vi "File Read Matrix.vi"(0 "file path (dialog if empty)":path, 11 "error in (no error)":errorcluster) -> (4 "Matrix":dbl[][](array[numeric]), 6 "Row Names":string[](array[string])=["AMP01BH", "AMP02AH", "AMP02BH", "AMP03AH", "AMP03BH", "AMP03CH", "AMP04AH", "AMP04BH", "AMP05AH", "AMP05BH", "AMP06AH", "AMP06BH", "AMP07AH", "AMP07BH", "AMP08AH", "AMP08BH", "AMP09AH", "AMP09BH", "AMP10AH", "AMP10BH", "AMU11AH", "AMU11BH", "AMP12AH", "AMP12BH", "AMP01AH", "AMP01BV", "AMP02AV", "AMP02BV", "AMP03AV", "AMP03BV", "AMP03CV", "AMP04AV", "AMP04BV", "AMP05AV", "AMP05BV", "AMP06AV", "AMP06BV", "AMP07AV", "AMP07BV", "AMP08AV", "AMP08BV", "AMP09AV", "AMP09BV", "AMP10AV", "AMP10BV", "AMU11AV", "AMU11BV", "AMP12AV", "AMP12BV", "AMP01AV"], 8 "Column Names":string[](array[string])=["ACH01B", "ACH02", "ACH03A", "ACH03B", "ACH04", "ACH05A", "ACH05B", "ACH06", "ACH07A", "ACH07B", "ACH08", "ACH09A", "ACH09B", "ACH10", "ACH11A", "ACH11B", "ACH12", "ACH01A", "ACV01B", "ALV02A", "ALV02B", "ACV03A", "ACV03B", "ALV04A", "ALV04B", "ACV05A", "ACV05B", "ALV06A", "ALV06B", "ACV07A", "ACV07B", "ALV08A", "ALV08B", "ACV09A", "ACV09B", "ALV10A", "ALV10B", "ACV11A", "ACV11B", "ALV12A", "ALV12B", "ACV01A"], 14 "Beam Energy (MeV)":dbl, 15 "error out":errorcluster)   [LabVIEW 2011, in "File VIs.lvlib"]
doc: "Reads a \"Response Matrix\" or \"Correction Matrix\" text file and converts the data to a 2D, double-precision array of numbers.\n\nFile format:\nFirst row: Beam Energy (MeV):<TAB>[Beam Energy Value for which the matrix was measured/calculated]\nSecond row*: Column names (Corrector names, for Response Matrix; BPM names, for Correction Matrix)\nAll other rows:\n Column 1: BPM names\n All other columns: Matrix value (mm/A, for Response Matrix; A/mm, for Correction Matrix)\nColumn separator: <TAB> character\n\n* The second row must begin with a <TAB> character\n\nEx.:\nBeam Energy (MeV):<TAB>1370\n<TAB>ACH01B<TAB>ACH02\nAMP01BH<TAB>5.10765701<TAB>-1.50432895\nAMP02AH<TAB>-0.41130998<TAB>0.95389896"
uses:
  File VIs.lvlib
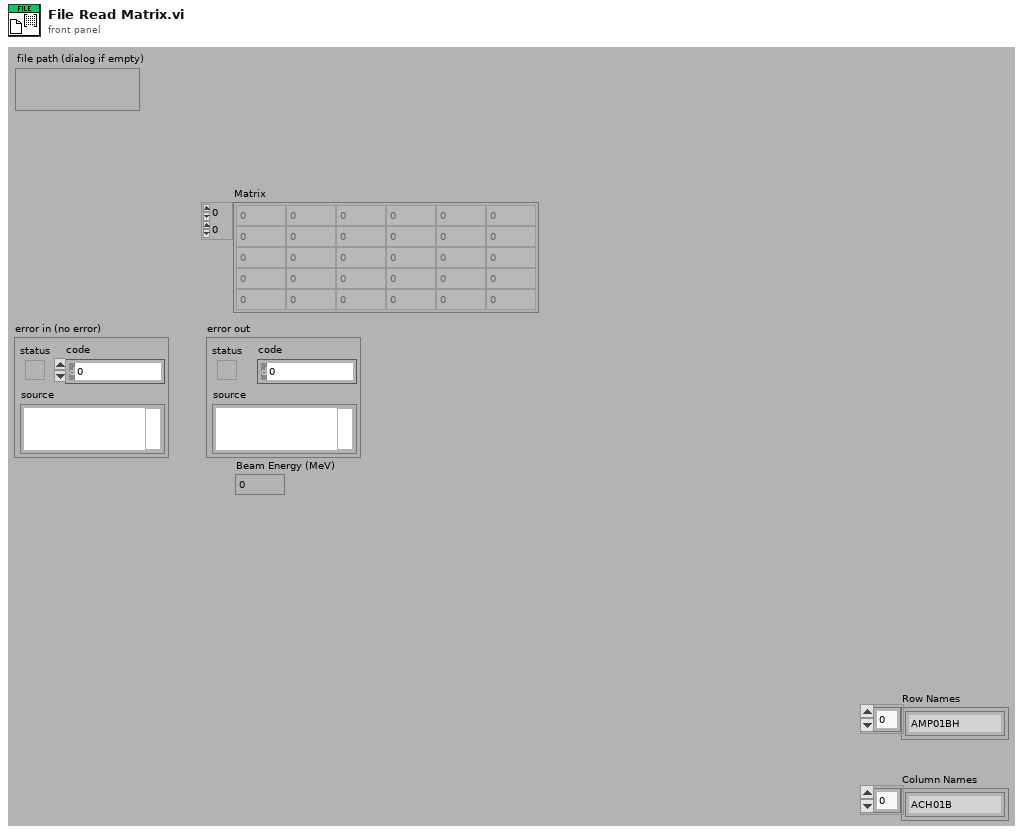
[diagram p1: front panel]
types:
  T1 = enum16{"open", "replace", "create", "open or create", "replace or create", "replace or create with confirmation"}
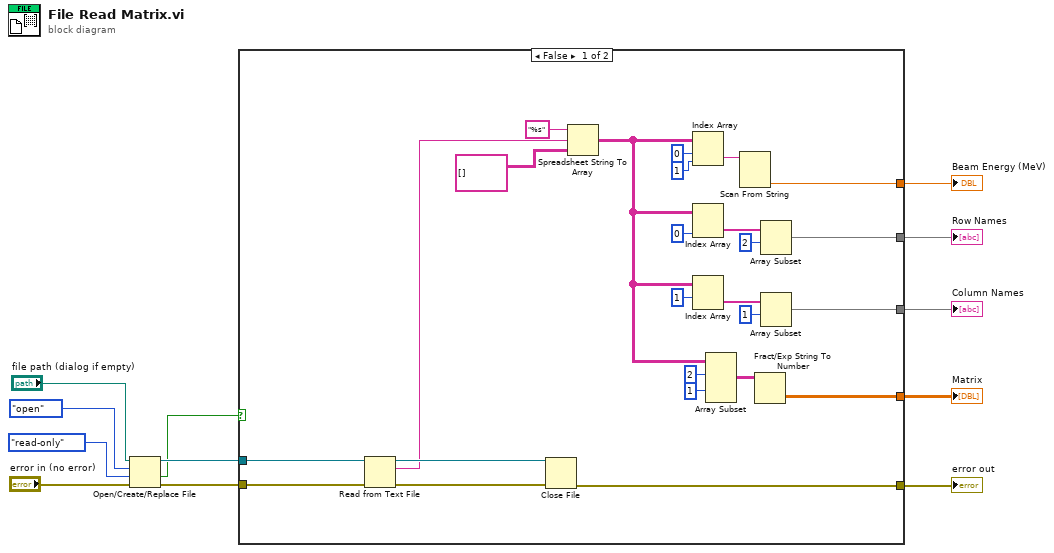
[diagram p0: block diagram]
diagram:
  n1 = Open/Create/Replace File(file path (use dialog)="file path (dialog if empty)", error in="error in (no error)", operation (0:open)=T1."open", access (0:read/write)=enum16{"read/write", "read-only", "write-only"}."read-only") -> (refnum out=w9:refnum<file>, cancelled=w4:bool, error out=w8:errorcluster)  [unwired: 2 in]
  n2 = case shown="False" w4 {
    tunnel: [w13 _] -> w12
    tunnel: w9 -> [w34 _]
    tunnel: w8 -> [w36 w38]
    tunnel: [w37 w38] -> w7
    tunnel: [w20 _] -> w3
    tunnel: [w19 _] -> w2
    tunnel: [w16 _] -> w1
    frame False {
      n3 = Read from Text File(file (use dialog)=w34, error in=w36) -> (refnum out=w33:refnum<file>, text=w25:string, error out=w35:errorcluster)  [unwired: 2 in, 1 out]
      n4 = Close File(refnum=w33, error in=w35) -> (error out=w37:errorcluster)  [unwired: 1 out]
      n5 = Spreadsheet String To Array(format string="%s", spreadsheet string=w25, array type (2D Dbl)=string[][] []) -> (array=w21:string[][])  [unwired: 1 in]
      n6 = Index Array(array=w21, index (row)=0, index (col)=1 ("disabled index (col)")) -> (element=w17:string)
      n7 = Index Array(array=w21, index (col)=0 ("index (row)")) -> (element=w28:string[])  [unwired: 1 in]
      n8 = Index Array(array=w21, index (row)=1 ("index (col)")) -> (element=w24:string[])  [unwired: 1 in]
      n9 = Array Subset(array=w21, index (row)=2 ("index"), index (col)=1 ("index")) -> (w32:string[][])  [unwired: 2 in]
      n10 = Scan From String(input string=w17) -> (output 1=w16:dbl)  [unwired: 4 in, 3 out]
      n11 = Fract/Exp String To Number(string=w32) -> (number=w13:dbl[][])  [unwired: 3 in, 1 out]
      n12 = Array Subset(array=w28, index=2) -> (w19:string[])  [unwired: 1 in]
      n13 = Array Subset(array=w24, index=1) -> (w20:string[])  [unwired: 1 in]
    }
    frame True {
    }
  }
  "error out" <- w7
  "Matrix" <- w12
  "Row Names" <- w2
  "Column Names" <- w3
  "Beam Energy (MeV)" <- w1
